vi "Get Current Resolution.vi"(11 "Current Rate in":dbl) -> (1 "Resolution in Digits":T1=5.5 caption="Current Resolution" items=["3 1/2"=3.5, "4 1/2"=4.5, "5 1/2"=5.5, "6 1/2"=6.5, "7 1/2"=7.5], 3 "Current Rate out":dbl)   [LabVIEW 2011, in "Switch-DMM Custom Device.lvlib"]
uses:
  Switch-DMM Custom Device.lvlib
  <instrlib>/niDMM/nidmm.llb/niDMM Resolution in Digits.ctl
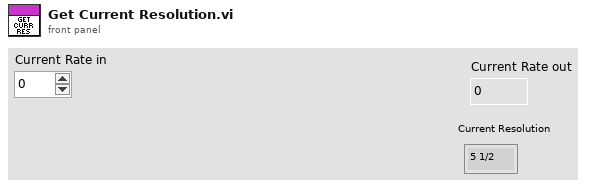
[diagram p1: front panel]
types:
  T1 = typedef "niDMM Resolution in Digits.ctl" = dbl
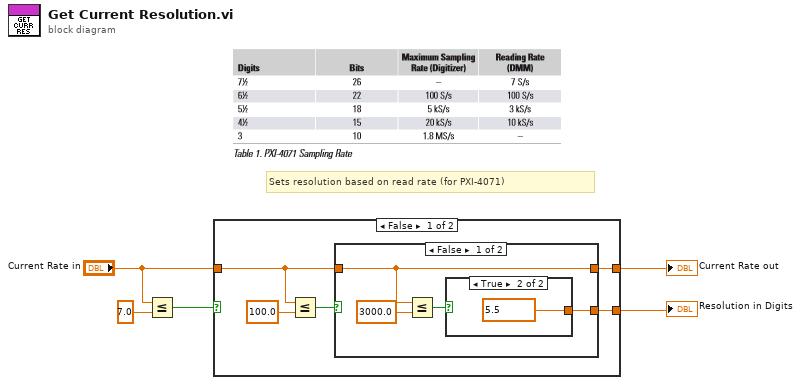
[diagram p0: block diagram]
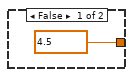
[diagram p2: hidden frame]
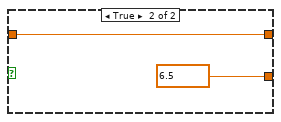
[diagram p3: hidden frame]
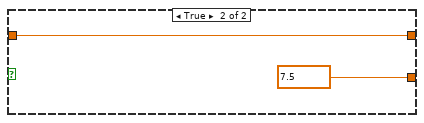
[diagram p4: hidden frame]
diagram:
  # "Sets resolution based on read rate (for PXI-4071)"
  n1 = Less Or Equal?(x="Current Rate in", y=7.0) -> (x <= y?=w4:bool)
  n2 = case shown="False" w4 {
    tunnel: "Current Rate in" -> [w7 w19]
    tunnel: [w8 w20] -> w2
    tunnel: [w6 w19] -> w1
    frame False {
      n3 = Less Or Equal?(x=w7, y=100.0) -> (x <= y?=w9:bool)
      n4 = case shown="False" w9 {
        tunnel: [w12 w18] -> w8
        tunnel: w7 -> [w11 w17]
        tunnel: [w11 w17] -> w6
        frame False {
          n5 = Less Or Equal?(x=w11, y=3000.0) -> (x <= y?=w13:bool)
          n6 = case shown="True" w13 {
            tunnel: [w15 w16] -> w12
            frame False {
              w15 = T1 4.5 items=["3 1/2"=3.5, "4 1/2"=4.5, "5 1/2"=5.5, "6 1/2"=6.5, "7 1/2"=7.5] ("Resolution in Digits")
            }
            frame True {
              w16 = T1 5.5 items=["3 1/2"=3.5, "4 1/2"=4.5, "5 1/2"=5.5, "6 1/2"=6.5, "7 1/2"=7.5] ("Resolution in Digits")
            }
          }
        }
        frame True {
          w18 = T1 6.5 items=["3 1/2"=3.5, "4 1/2"=4.5, "5 1/2"=5.5, "6 1/2"=6.5, "7 1/2"=7.5] ("Resolution in Digits")
        }
      }
    }
    frame True {
      w20 = T1 7.5 items=["3 1/2"=3.5, "4 1/2"=4.5, "5 1/2"=5.5, "6 1/2"=6.5, "7 1/2"=7.5] ("Resolution in Digits")
    }
  }
  "Current Rate out" <- w1
  "Resolution in Digits" <- w2
